vi "Target Refresh Tracker.vi"(8 "Error In":errorcluster, 11 "Progress bar (auto closed)":refnum<vi>) -> ()   [LabVIEW 2019, in "Project.Dependencies Finder.lvlib"]
doc: "Tracks target refresh progress. Stop VI using 'Stop Target Refresh.vi'\n\n2020-12-07: Henrik Dueholm Hansen"
uses:
  Project.Dependencies Finder.lvlib
panel:
  out "Target":i32
  out "Progress":i32
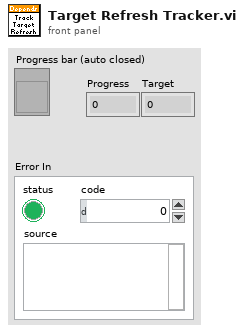
[diagram p1: front panel]
types:
  T1 = typedef "Project.Dependencies Finder.lvlib/Ctl_Progress Queue.ctl" = refnum<queue>
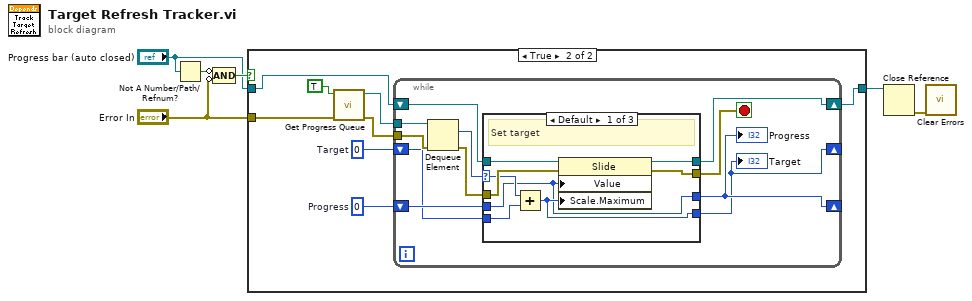
[diagram p0: block diagram]
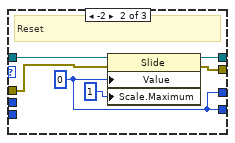
[diagram p3: hidden frame]
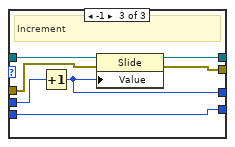
[diagram p4: hidden frame]
diagram:
  n1 = Not A Number/Path/Refnum?(number/path/refnum="Progress bar (auto closed)") -> (NaN/Path/Refnum?=w6:bool)
  n2 = Compound Arithmetic op=AND(invert w6, invert "Error In") -> (w5:bool)
  n3 = case shown="True" w5 {
    tunnel: "Error In" -> [_ w15]
    tunnel: "Progress bar (auto closed)" -> [w7 w12]
    tunnel: [w7 w10] -> w2
    frame False {
    }
    frame True {
      w8 = 0  # Target
      w13 = 0  # Progress
      n4 = call "Get Progress Queue.vi"("error in"=w15, "Enable Tracking?"=TRUE) -> ("error out"=w11:errorcluster, "Progress queue"=w14:T1)  [unwired: 8 in]
      n5 = while {
        tunnel: w14 -> [w26]
        shift-right: [w24] -> _
        shift-left: w13 -> [w25]
        shift-right: [w18] -> w10
        shift-left: w12 -> [w23]
        tunnel: w11 -> [w19]
        shift-right: [w16] -> _
        shift-left: w8 -> [w17]
        stop <- w21 stop-if-true
        n6 = Dequeue Element(queue=w26, error in (no error)=w19) -> (element=w20:i32, error out=w22:errorcluster)  [unwired: 1 in, 2 out]
        n7 = case shown="Default" w20 {
          selector: w20 -> [w29 _ _]
          tunnel: w25 -> [w27 _ w47]
          tunnel: [w27 w39 w45] -> w24
          tunnel: w23 -> [w34 w40 w46]
          tunnel: w22 -> [w32 w37 w44]
          tunnel: [w31 w36 w43] -> w21
          tunnel: [w33 w38 w42] -> w18
          tunnel: w17 -> [w30 _ w41]
          tunnel: [w28 w39 w41] -> w16
          frame Default {
            # "Set target"
            n8 = Add(x=w29, y=w30) -> (x+y=w28:i32)
            n9 = property class="Slide"(reference=w34, error in=w32, "Value"=w27, "Scale.Maximum"=w28) -> (reference out=w33:refnum<vi>, error out=w31:errorcluster)
          }
          frame -2 {
            w39 = 0
            # "Reset"
            n10 = property class="Slide"(reference=w40, error in=w37, "Value"=w39, "Scale.Maximum"=1) -> (reference out=w38:refnum<vi>, error out=w36:errorcluster)
          }
          frame -1 {
            # "Increment"
            n11 = Increment(x=w47) -> (x+1=w45:i32)
            n12 = property class="Slide"(reference=w46, error in=w44, "Value"=w45) -> (reference out=w42:refnum<vi>, error out=w43:errorcluster)
          }
        }
        "Progress" <- w24
        "Target" <- w16
      }
    }
  }
  n13 = Close Reference(reference=w2) -> (error out=w1:errorcluster)  [unwired: 1 in]
  n14 = call <vilib>:"Clear Errors.vi"("error in (no error)"=w1) -> ()  [unwired: 5 in, 2 out]
